vi "PRAT Read All MW100 Inputs.vi"(0 "MW100":refnum<visa-resource-name>="MW100", 1 "LV Program":T1, 11 "Error In":errorcluster) -> (4 "dup VISA session":refnum<visa-resource-name>, 6 "Data (Label, Channel, Data)":string[][](array[string]), 10 "PowerData":T2, 15 "error out":errorcluster)   [LabVIEW 2020]
uses:
  Type Definitions/HEWH Power Data.ctl
  Utility/Save File/File Setup (Public)/Type Definition/Save File DOE LabView Program.ctl
  Type Definitions/PRAT Channel Settings.ctl
  Utility/Save File/File Setup.lvlib
panel:
  out "Channel List":string[](array[string])
  out "All Data":dbl[](array[numeric]) format="%.4f"
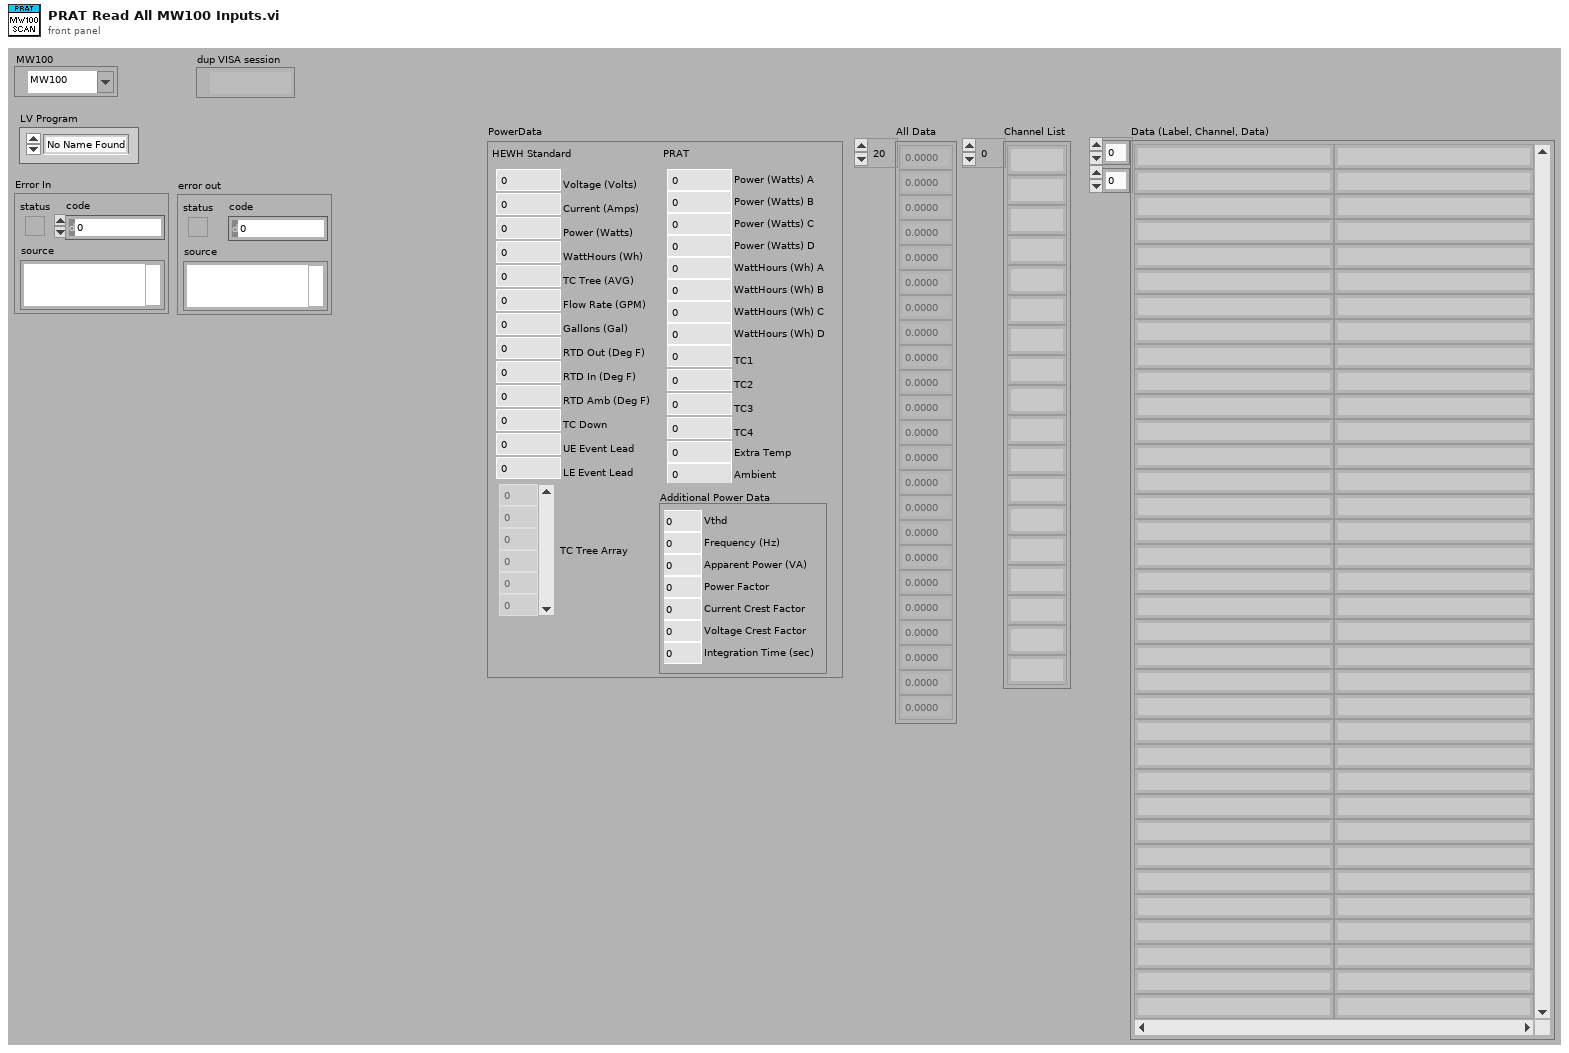
[diagram p1: front panel]
types:
  T1 = typedef "File Setup.lvlib/Save File DOE LabView Program.ctl" = enum16{"No Name Found", "DOE Stand", "Dishwasher Kitchen", "Portable Stand", "HEWH", "Dryer", "Dryer WILT", "HCC", "PRAT", "HEWH RLT", "Refrigeration", "Gas Water Heater"}
  T2 = typedef "HEWH Power Data.ctl" = cluster{"HEWH Standard":cluster{"Voltage (Volts)":dbl, "Current (Amps)":dbl, "Power (Watts)":dbl, "WattHours (Wh)":dbl, "TC Tree (AVG)":dbl, "Flow Rate (GPM)":dbl, "Gallons (Gal)":dbl, "RTD Out (Deg F)":dbl, "RTD In (Deg F)":dbl, "RTD Amb (Deg F)":dbl, "TC Down":dbl, "UE Event Lead":i32, "LE Event Lead":i32, "TC Tree Array":dbl[]}, "PRAT":cluster{"Power (Watts) A":dbl, "Power (Watts) B":dbl, "Power (Watts) C":dbl, "Power (Watts) D":dbl, "TC1":dbl, "TC2":dbl, "TC3":dbl, "TC4":dbl, "WattHours (Wh) A":dbl, "WattHours (Wh) B":dbl, "WattHours (Wh) C":dbl, "WattHours (Wh) D":dbl, "Ambient":dbl, "Extra Temp":dbl}, "Additional Power Data":cluster{"Vthd":dbl, "Frequency (Hz)":dbl, "Apparent Power (VA)":dbl, "Power Factor":dbl, "Current Crest Factor":dbl, "Voltage Crest Factor":dbl, "Integration Time (sec)":dbl}}
  T3 = typedef "PRAT Channel Settings.ctl" = string
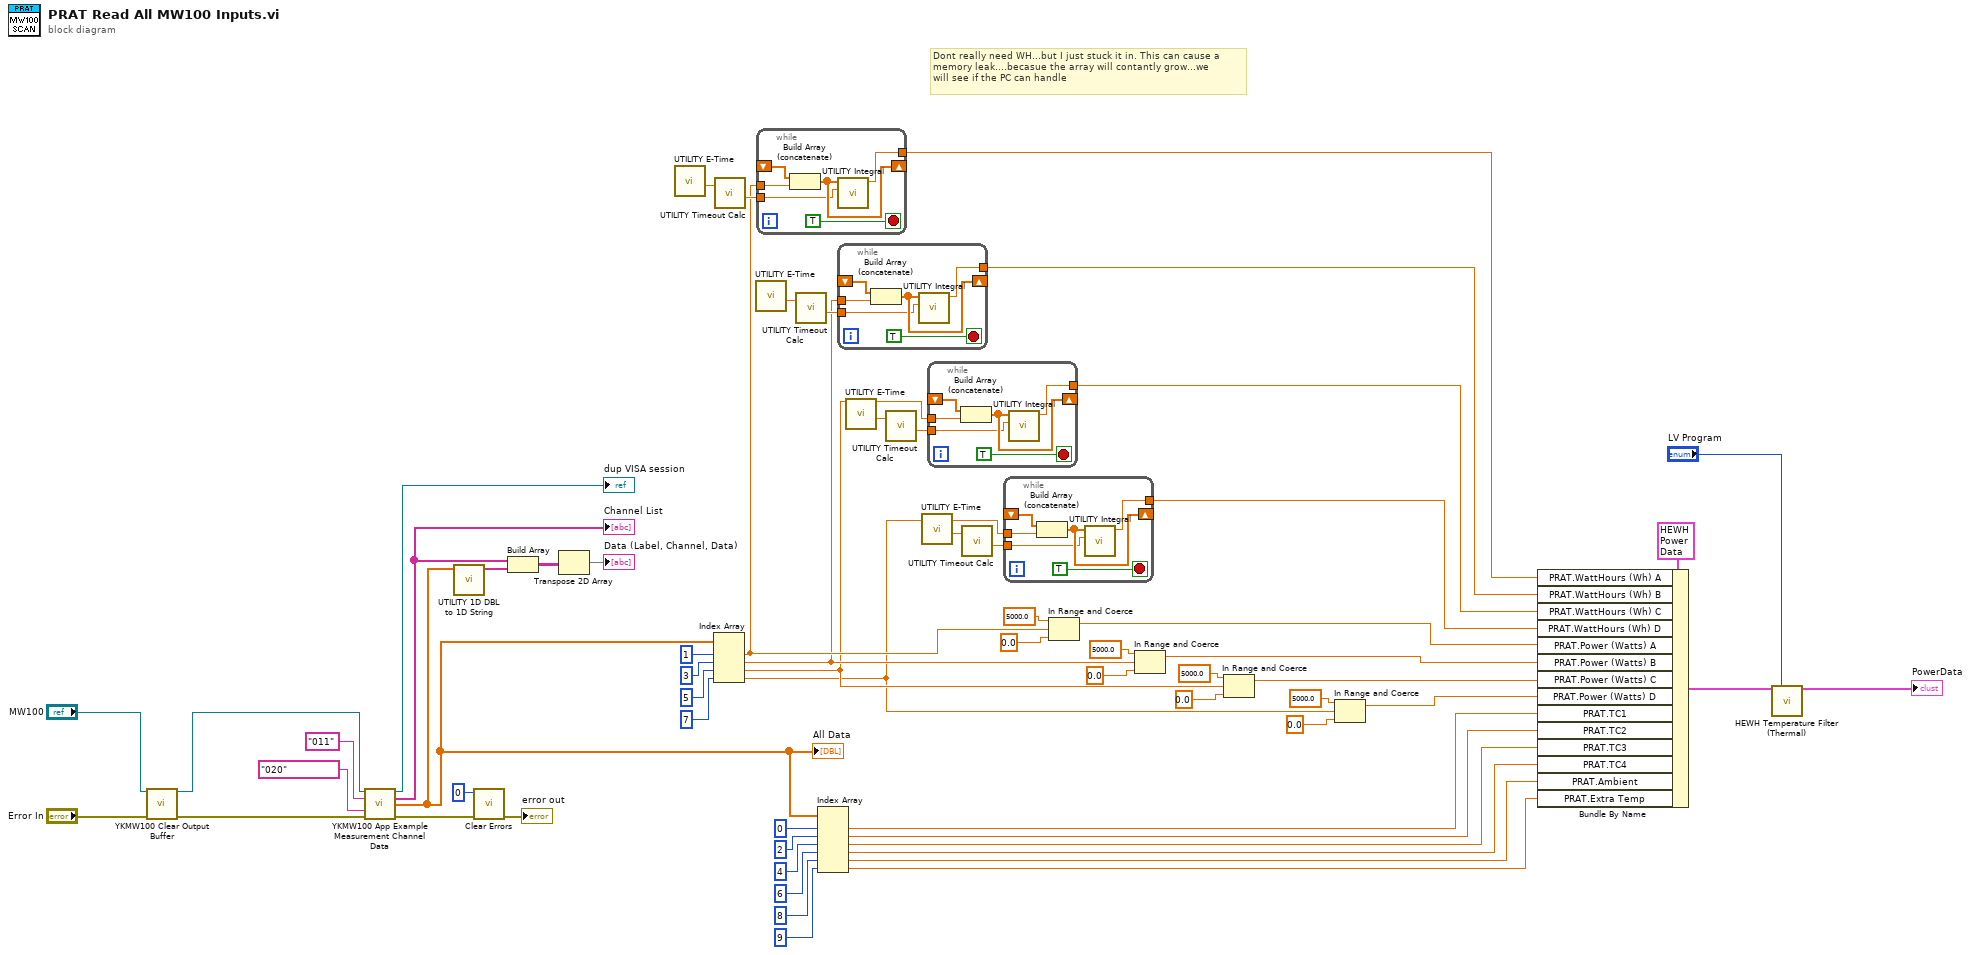
[diagram p0: block diagram]
diagram:
  # "Dont really need WH...but I just stuck it in. This can cause a \nmemory leak....becasue the array will contantly grow...we \nwill see if the PC can handle"
  n1 = call "YKMW100 Clear Output Buffer.vi"("VISA session"="MW100", "error in (no error)"="Error In") -> ("dup VISA session"=w2:refnum<visa-resource-name>, "error out"=w4:errorcluster)  [unwired: 12 in]
  n2 = call "YKMW100 App Example Measurement Channel Data.vi"("VISA session"=w2, "Start Channel (001)"=T3 "011" ("PRAT Channels"), "End Channel (001)"=T3 "020" ("PRAT Channels"), "error in (no error)"=w4) -> ("dup VISA session"=→"dup VISA session":refnum<visa-resource-name>, "Channel List"=w29:string[], "Data List"=w28:dbl[], "error out"=w43:errorcluster)  [unwired: 4 in, 4 out]
  "All Data" <- w28
  "Channel List" <- w29
  n3 = call "UTILITY 1D DBL to 1D String.vi"("1D DBL"=w28) -> ("1D String"=w27:string[])  [unwired: 10 in]
  n4 = call <vilib>:"Clear Errors.vi"("error in (no error)"=w43, "specific error code to clear (0: all)"=0) -> ("error out"=→"error out":errorcluster)  [unwired: 4 in, 1 out]
  n5 = Build Array(w29, w27) -> (w26:string[][])
  n6 = Transpose 2D Array(2D array=w26) -> (transposed array=→"Data (Label, Channel, Data)":string[][])
  n7 = call "UTILITY E-Time.vi"() -> ("Elapsed Time (sec)"=w41:dbl)  [unwired: 9 in, 2 out]
  n8 = Index Array(array=w28, index #1=1 ("index"), index #2=3 ("index"), index #3=5 ("index"), index #4=7 ("index")) -> (element #1=w22:dbl, element #2=w19:dbl, element #3=w14:dbl, element #4=w10:dbl)
  n9 = call "UTILITY Timeout Calc.vi"("Timer"=w41) -> ("Rate"=w40:dbl)  [unwired: 9 in, 1 out]
  n10 = call "UTILITY E-Time.vi"() -> ("Elapsed Time (sec)"=w37:dbl)  [unwired: 9 in, 2 out]
  n11 = while {
    shift-right: [w68] -> _
    shift-left: _ -> [w69]
    tunnel: w40 -> [w67]
    tunnel: [w66] -> w39
    tunnel: w22 -> [w65]
    stop <- TRUE stop-if-true
    n12 = Build Array (concatenate)(w69, w65) -> (w68:dbl[])
    n13 = call "UTILITY Integral.vi"("dt"=w67, "Array Input"=w68) -> ("Integral"=w66:dbl)  [unwired: 8 in, 1 out]
  }
  n14 = call "UTILITY Timeout Calc.vi"("Timer"=w37) -> ("Rate"=w38:dbl)  [unwired: 9 in, 1 out]
  n15 = Index Array(array=w28, index #1=0 ("index"), index #2=2 ("index"), index #3=4 ("index"), index #4=6 ("index"), index #5=8 ("index"), index #6=9 ("index")) -> (element #1=w58:dbl, element #2=w57:dbl, element #3=w56:dbl, element #4=w55:dbl, element #5=w45:dbl, element #6=w44:dbl)
  n16 = while {
    shift-right: [w74] -> _
    shift-left: _ -> [w75]
    tunnel: w38 -> [w73]
    tunnel: [w72] -> w36
    tunnel: w19 -> [w71]
    stop <- TRUE stop-if-true
    n17 = Build Array (concatenate)(w75, w71) -> (w74:dbl[])
    n18 = call "UTILITY Integral.vi"("dt"=w73, "Array Input"=w74) -> ("Integral"=w72:dbl)  [unwired: 8 in, 1 out]
  }
  n19 = call "UTILITY E-Time.vi"() -> ("Elapsed Time (sec)"=w35:dbl)  [unwired: 9 in, 2 out]
  n20 = call "UTILITY Timeout Calc.vi"("Timer"=w35) -> ("Rate"=w34:dbl)  [unwired: 9 in, 1 out]
  n21 = call "UTILITY E-Time.vi"() -> ("Elapsed Time (sec)"=w32:dbl)  [unwired: 9 in, 2 out]
  n22 = while {
    shift-right: [w80] -> _
    shift-left: _ -> [w81]
    tunnel: w34 -> [w79]
    tunnel: [w78] -> w31
    tunnel: w14 -> [w77]
    stop <- TRUE stop-if-true
    n23 = Build Array (concatenate)(w81, w77) -> (w80:dbl[])
    n24 = call "UTILITY Integral.vi"("dt"=w79, "Array Input"=w80) -> ("Integral"=w78:dbl)  [unwired: 8 in, 1 out]
  }
  n25 = call "UTILITY Timeout Calc.vi"("Timer"=w32) -> ("Rate"=w33:dbl)  [unwired: 9 in, 1 out]
  n26 = while {
    shift-right: [w86] -> _
    shift-left: _ -> [w87]
    tunnel: w33 -> [w85]
    tunnel: [w84] -> w30
    tunnel: w10 -> [w83]
    stop <- TRUE stop-if-true
    n27 = Build Array (concatenate)(w87, w83) -> (w86:dbl[])
    n28 = call "UTILITY Integral.vi"("dt"=w85, "Array Input"=w86) -> ("Integral"=w84:dbl)  [unwired: 8 in, 1 out]
  }
  n29 = In Range and Coerce(upper limit=5000.0, x=w22, lower limit=0.0) -> (coerced(x)=w21:dbl)  [unwired: 1 out]
  n30 = In Range and Coerce(upper limit=5000.0, x=w19, lower limit=0.0) -> (coerced(x)=w17:dbl)  [unwired: 1 out]
  n31 = In Range and Coerce(upper limit=5000.0, x=w14, lower limit=0.0) -> (coerced(x)=w13:dbl)  [unwired: 1 out]
  n32 = In Range and Coerce(upper limit=5000.0, x=w10, lower limit=0.0) -> (coerced(x)=w9:dbl)  [unwired: 1 out]
  n33 = Bundle By Name(cluster=T2 {"HEWH Standard"={"Voltage (Volts)"=240.0, "Current (Amps)"=0.017575, "Power (Watts)"=4.218, "WattHours (Wh)"=19682.0, "TC Tree (AVG)"=0.0, "Flow Rate (GPM)"=0.0, "Gallons (Gal)"=0.0, "RTD Out (Deg F)"=0.0, "RTD In (Deg F)"=0.0, "RTD Amb (Deg F)"=0.0, "TC Down"=0.0, "UE Event Lead"=0, "LE Event Lead"=0, "TC Tree Array"=[]}, "PRAT"={"Power (Watts) A"=4192.0, "Power (Watts) B"=4192.0, "Power (Watts) C"=4192.0, "Power (Watts) D"=4192.0, "TC1"=0.0, "TC2"=0.0, "TC3"=0.0, "TC4"=0.0, "WattHours (Wh) A"=4192.0, "WattHours (Wh) B"=4192.0, "WattHours (Wh) C"=4192.0, "WattHours (Wh) D"=4192.0, "Ambient"=0.0, "Extra Temp"=0.0}, "Additional Power Data"={"Vthd"=236.2, "Frequency (Hz)"=236.2, "Apparent Power (VA)"=236.2, "Power Factor"=236.2, "Current Crest Factor"=236.2, "Voltage Crest Factor"=236.2, "Integration Time (sec)"=236.2}} ("PowerData 2"), "PRAT.WattHours (Wh) A"=w39, "PRAT.WattHours (Wh) B"=w36, "PRAT.WattHours (Wh) C"=w31, "PRAT.WattHours (Wh) D"=w30, "PRAT.Power (Watts) A"=w21, "PRAT.Power (Watts) B"=w17, "PRAT.Power (Watts) C"=w13, "PRAT.Power (Watts) D"=w9, "PRAT.TC1"=w58, "PRAT.TC2"=w57, "PRAT.TC3"=w56, "PRAT.TC4"=w55, "PRAT.Ambient"=w45, "PRAT.Extra Temp"=w44) -> (w8:T2)
  n34 = call "HEWH Temperature Filter (Thermal).vi"("HEWH Data"=w8, "LV Program"="LV Program") -> ("HEWH Data Out"=→"PowerData":T2)  [unwired: 12 in, 1 out]
